vi "SRQ Wait TEST.vi"(2 "error out":errorcluster, 3 "VISA GPIB Resource":refnum<visa-resource-name>) -> (0 "error out 2":errorcluster, 1 "VISA GPIB Resource 2":refnum<visa-resource-name>)   [LabVIEW 2018]
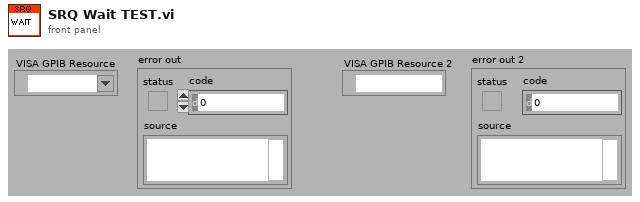
[diagram p1: front panel]
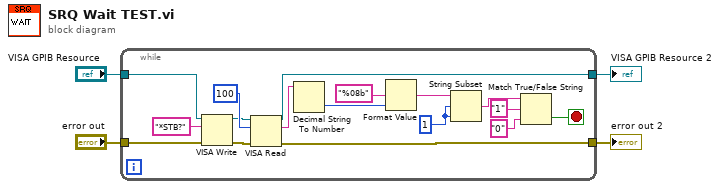
[diagram p0: block diagram]
diagram:
  n1 = while {
    tunnel: [w11] -> w1
    tunnel: [w10] -> w2
    tunnel: "VISA GPIB Resource" -> [w6]
    tunnel: "error out" -> [w5]
    stop <- w9 stop-if-true
    w7 = 1
    n2 = VISA Write(VISA resource name=w6, write buffer="*STB?", error in (no error)=w5) -> (VISA resource name out=w13:refnum<visa-resource-name>, error out=w12:errorcluster)  [unwired: 1 out]
    n3 = VISA Read(VISA resource name=w13, byte count=100, error in (no error)=w12) -> (VISA resource name out=w11:refnum<visa-resource-name>, read buffer=w16:string, error out=w10:errorcluster)  [unwired: 1 out]
    n4 = Decimal String To Number(string=w16) -> (number=w17:i32)  [unwired: 3 out]
    n5 = Format Value(format string="%08b", value (0)=w17) -> (output string=w19:string)  [unwired: 1 out]
    n6 = String Subset(string=w19, offset (0)=w7, length (rest)=w7) -> (substring=w20:string)
    n7 = Match True/False String(2:"0", 3:"1", 4:w20) -> (0:w9:bool)  [unwired: 1 out]
  }
  "error out 2" <- w2
  "VISA GPIB Resource 2" <- w1
